vi "UICtrls_BuildMessage_(poly).vi"   [LabVIEW 2025]
uses:
  UI_Manager.lvlib
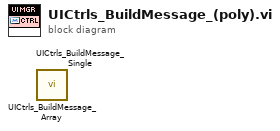
[diagram p0: block diagram]
diagram:
  n1 = call "UICtrls_BuildMessage_Array.vi"() -> ()  [unwired: 7 in, 2 out]
  n2 = call "UICtrls_BuildMessage_Single.vi"() -> ()  [unwired: 7 in, 2 out]
